vi "GetScriptStringForDisplay.vi"(10 "Script":string[](array[string]), 11 "INI File Path":path) -> (3 "Script String":string)   [LabVIEW 2018]
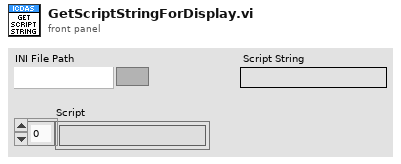
[diagram p1: front panel]
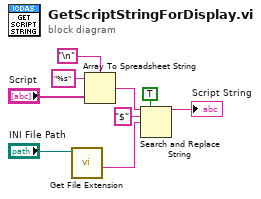
[diagram p0: block diagram]
diagram:
  n1 = call <vilib>:"Get File Extension.vi"("file"="INI File Path") -> ("filename without extension"=w7:string)  [unwired: 6 in, 4 out]
  n2 = Array To Spreadsheet String(delimiter (Tab)="\n", array="Script", 3:"%s" ("format string")) -> (spreadsheet string=w5:string)
  n3 = Search and Replace String(replace all?=TRUE ("replace all? (F)"), input string=w5, search string="$", replace string=w7) -> (result string=→"Script String":string)  [unwired: 4 in, 3 out]
